vi "Set Switch Cooling Time.vi"(2 "error in":T1, 3 "Switch Cooling Time (sec)":dbl=15.0 min=5.0 max=120.0, 4 "connection ID":refnum<visa-resource-name>) -> (0 "error out":T1, 1 "connection ID out":refnum<visa-resource-name>)   [LabVIEW 2019]
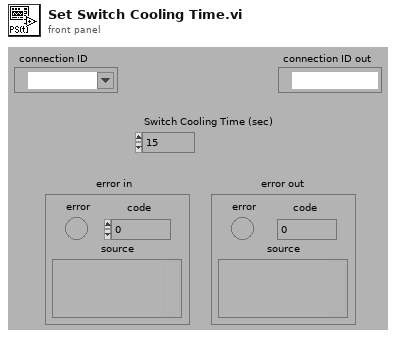
[diagram p1: front panel]
types:
  T1 = cluster{"error":bool, "code":i32, "source":string}
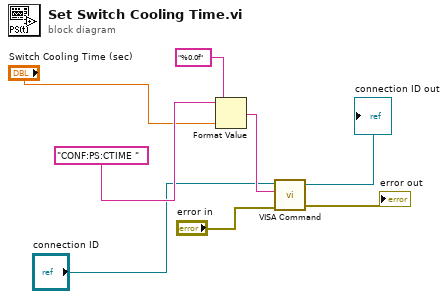
[diagram p0: block diagram]
diagram:
  n1 = Format Value(string ("")="CONF:PS:CTIME ", format string="%0.0f", value (0)="Switch Cooling Time (sec)") -> (output string=w5:string)
  n2 = call "VISA Command.vi"("error in (no error)"="error in", "Command"=w5, "VISA resource name"="connection ID") -> ("error out"=→"error out":errorcluster, "VISA resource name out"=→"connection ID out":refnum<visa-resource-name>)  [unwired: 1 in, 1 out]
